vi "Exemple_Preprocessing_scale.vi"() -> ()   [LabVIEW 2020]
panel:
  out "Data":T1
  out "error out":errorcluster
  in  "X":string[][](array[string])=[["0", "0"], ["0", "0"], ["1", "1"], ["1", "1"]]
  in  "error in":errorcluster caption="entrée d'erreur"
  in  "scale":T2={"axis"=0, "with_mean"=TRUE, "with_std"=TRUE, "copy"=TRUE}
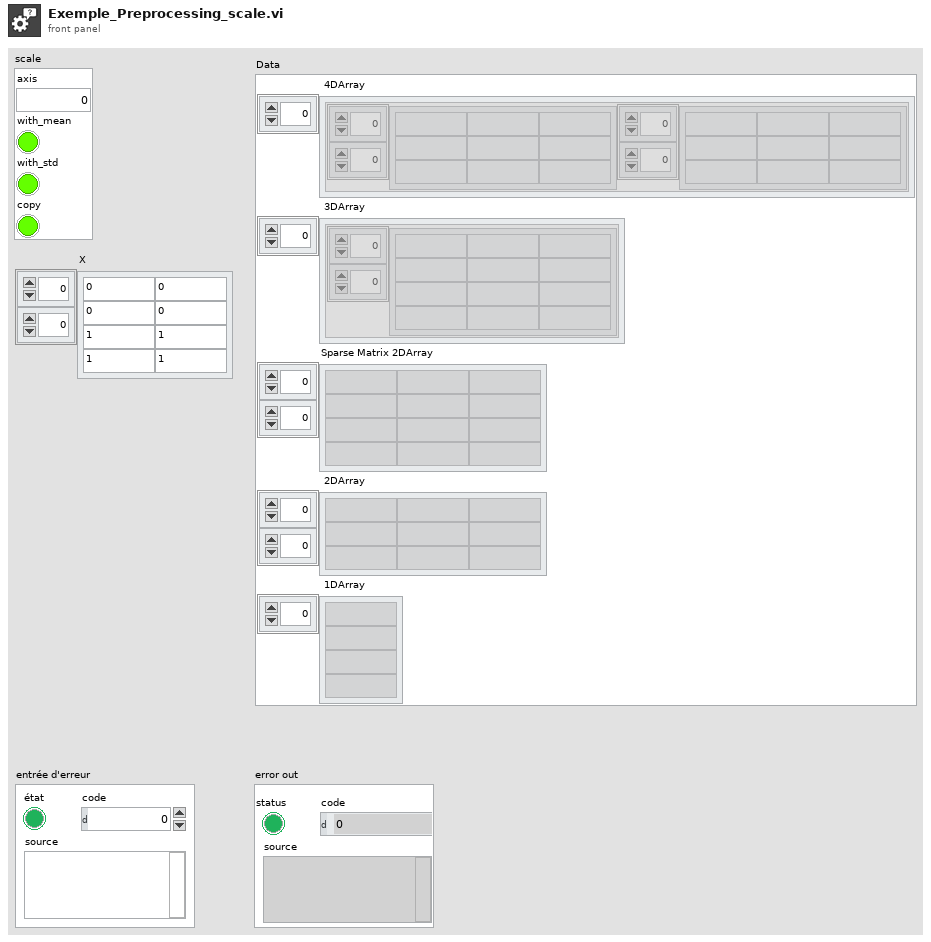
[diagram p1: front panel]
types:
  T1 = cluster{" 4DArray":cluster{"1":string[][], "2":string[][]}[], " 3DArray":cluster{"Tableau":string[][]}[], "Sparse Matrix 2DArray":string[][], " 2DArray":string[][], " 1DArray":string[]}
  T2 = cluster{"axis":i32, "with_mean":bool, "with_std":bool, "copy":bool}
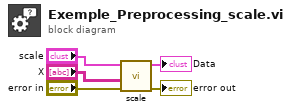
[diagram p0: block diagram]
diagram:
  n1 = call "scale.vi"("error in"="error in", "X"="X", "scale"="scale") -> ("error out"=→"error out":errorcluster, "Data"=→"Data":T1)  [unwired: 7 in]
